vi "MainApp.vi"() -> ()   [LabVIEW 2018]
panel:
  out "Error Out":errorcluster
  in  "Plots":T1(tab)
  out "EEG":cluster{dbl[], dbl[]}(graph)
  out "PS":cluster{dbl[], dbl[]}(graph)
  out "Filtered":cluster{dbl[], dbl[]}(graph)
  in  "Save":bool
  in  "Filename":string
  out "Value":dbl
  out "State":T2(ring)
  in  "Stop":bool
  in  "Start":bool
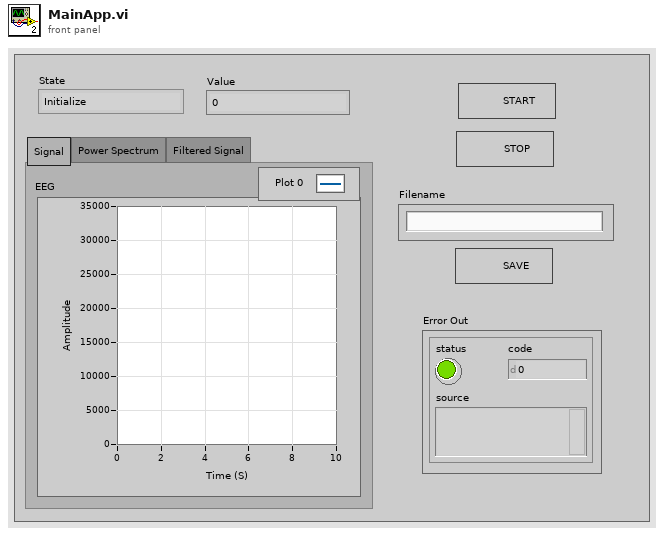
[diagram p1: front panel]
types:
  T1 = enum32{"Signal", "Power Spectrum", "Filtered Signal"}
  T2 = enum16{"Initialize", "Standby", "Record Data", "Filter Signal", "Save to File", "Stop"}
  T3 = enum16{"Standard", "Buffered", "CRLF", "Immediate"}
  T4 = enum16{"open", "replace", "create", "open or create", "replace or create", "replace or create with confirmation"}
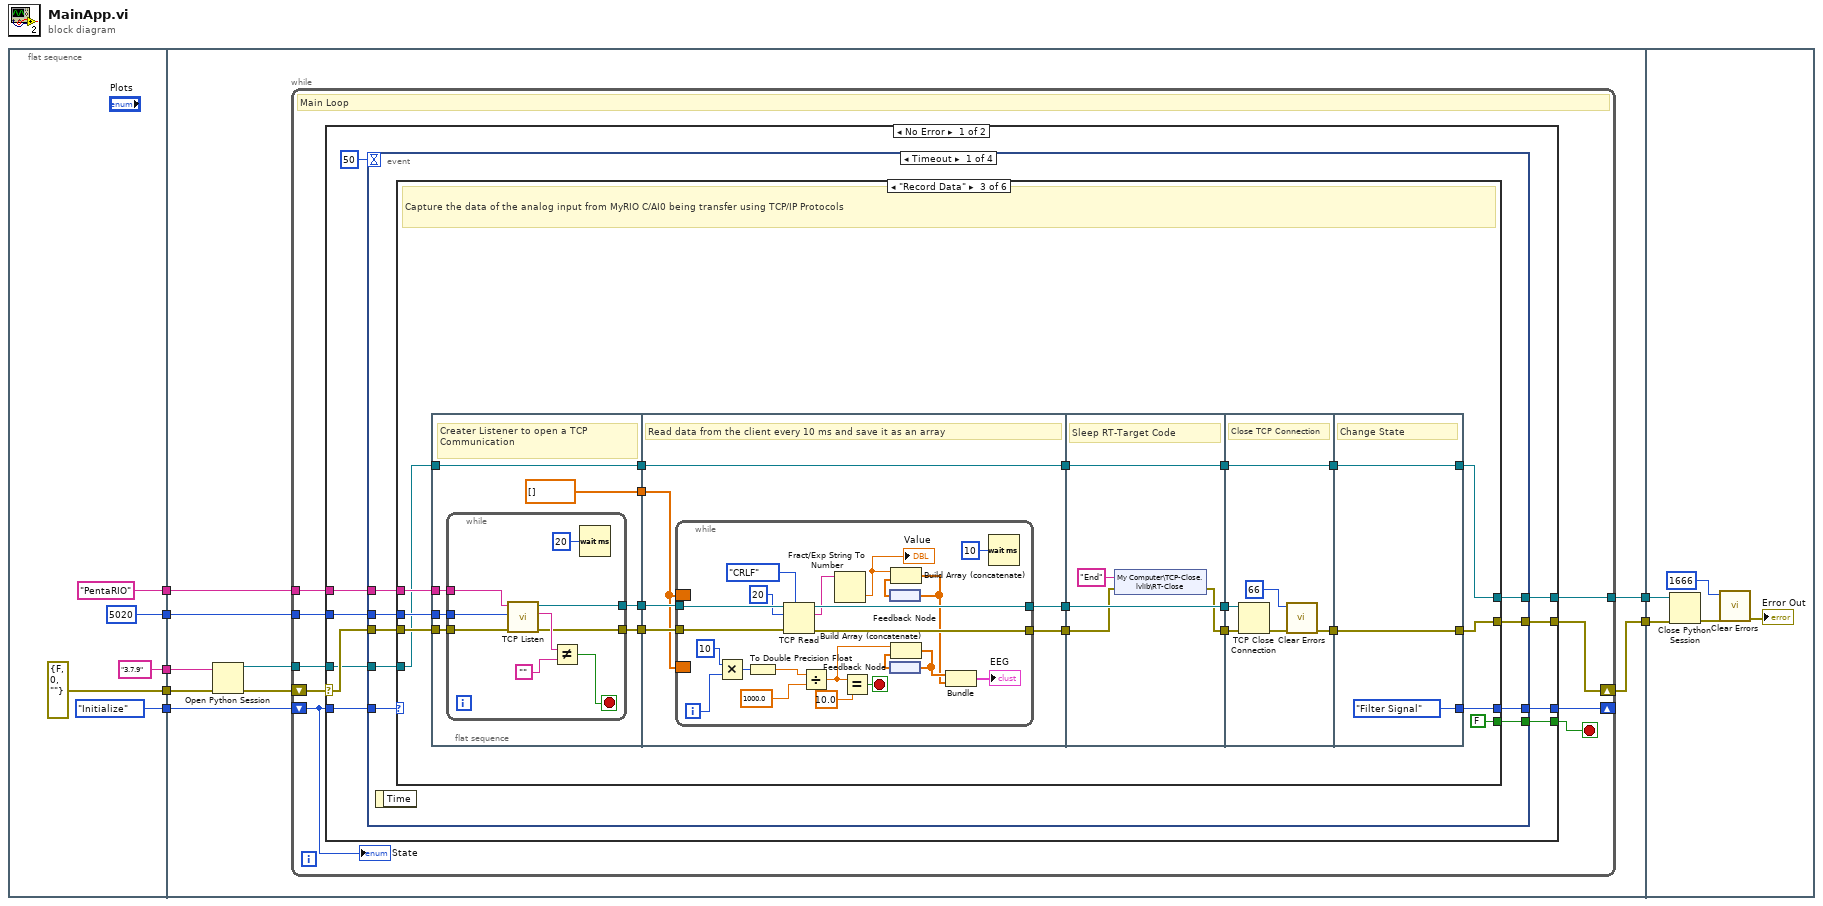
[diagram p0: block diagram]
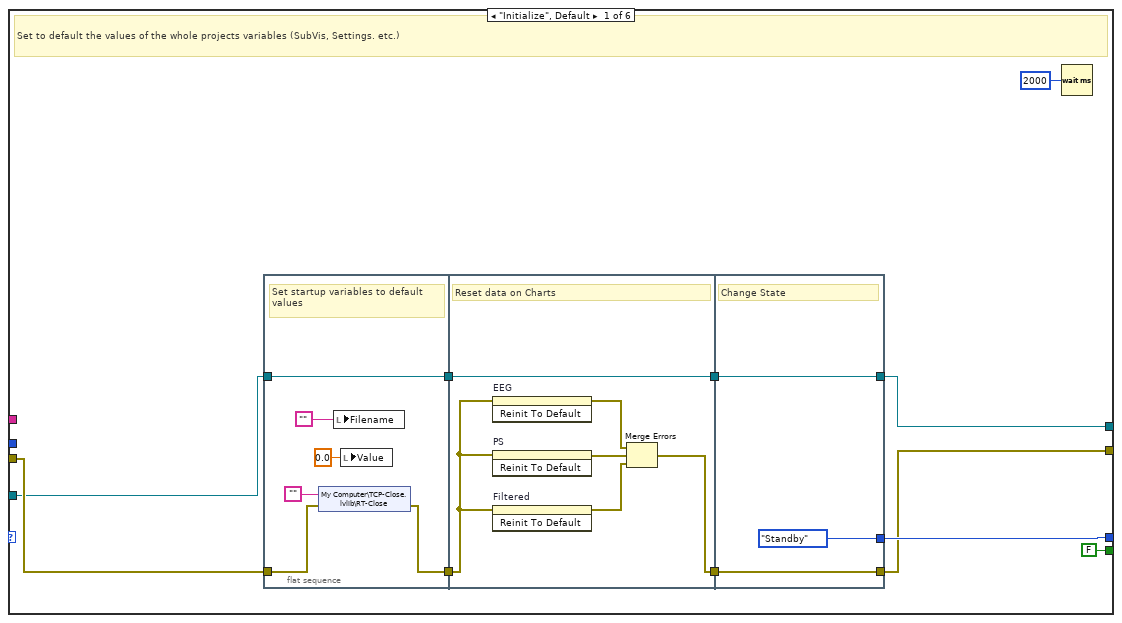
[diagram p2: hidden frame]
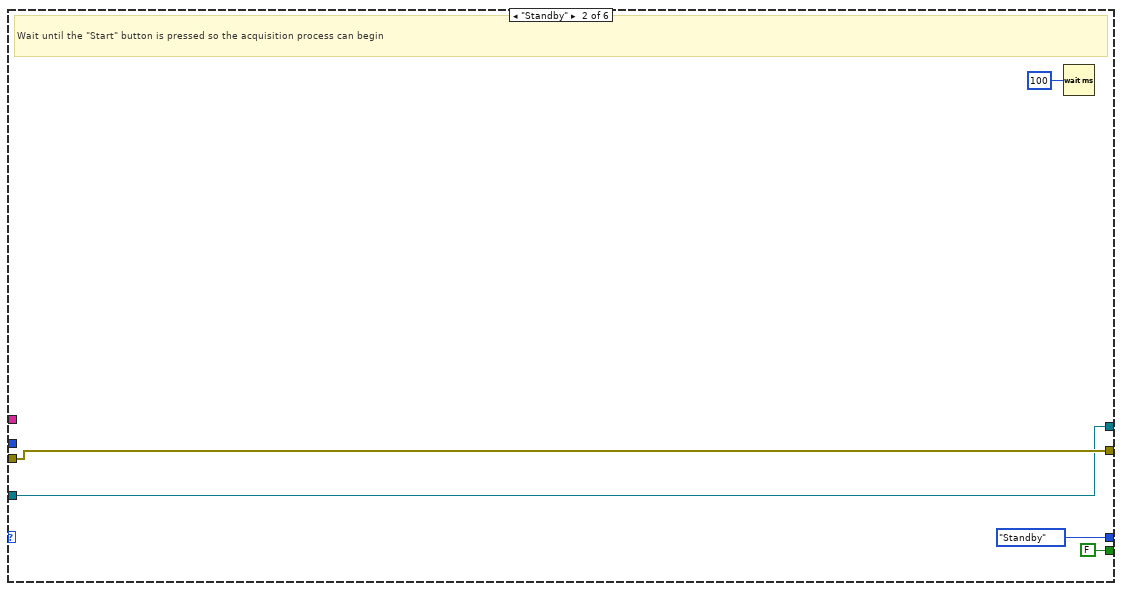
[diagram p3: hidden frame]
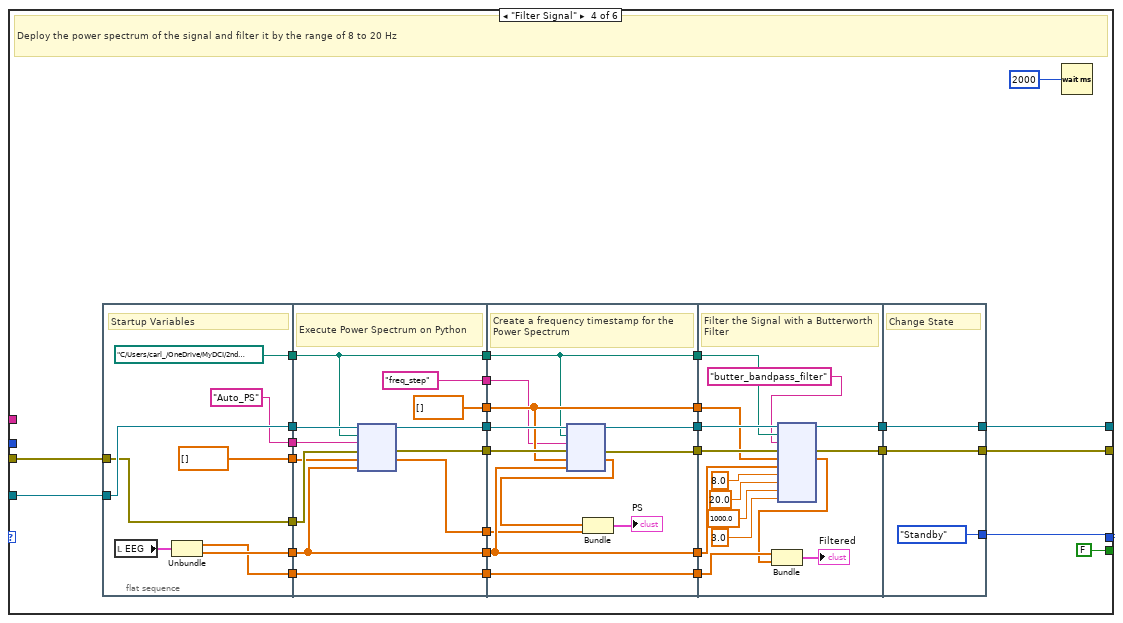
[diagram p4: hidden frame]
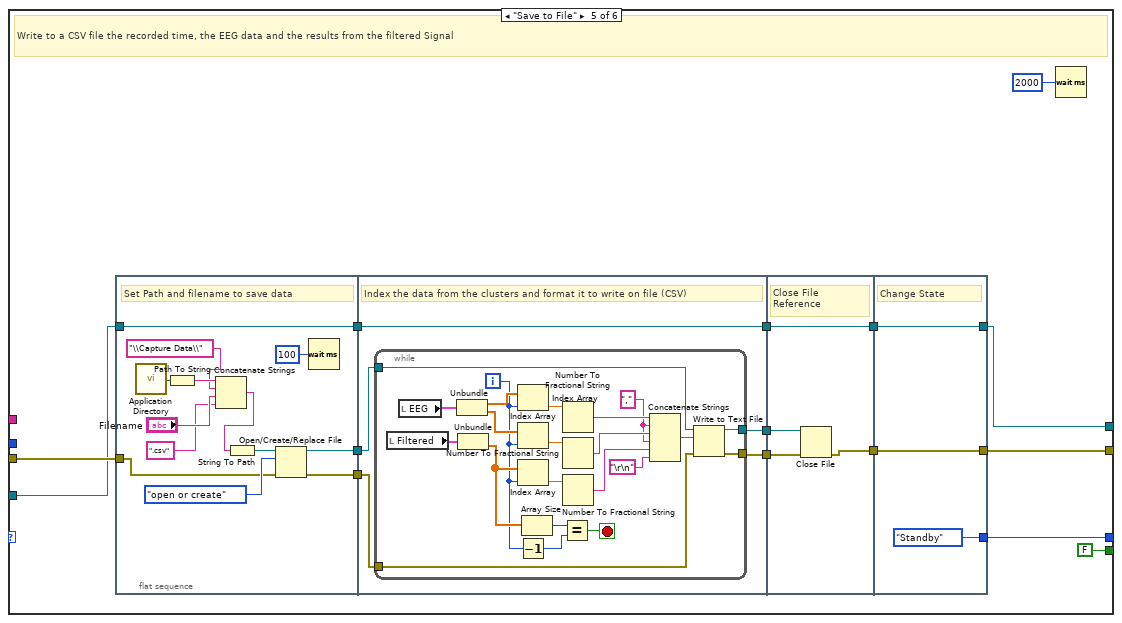
[diagram p5: hidden frame]
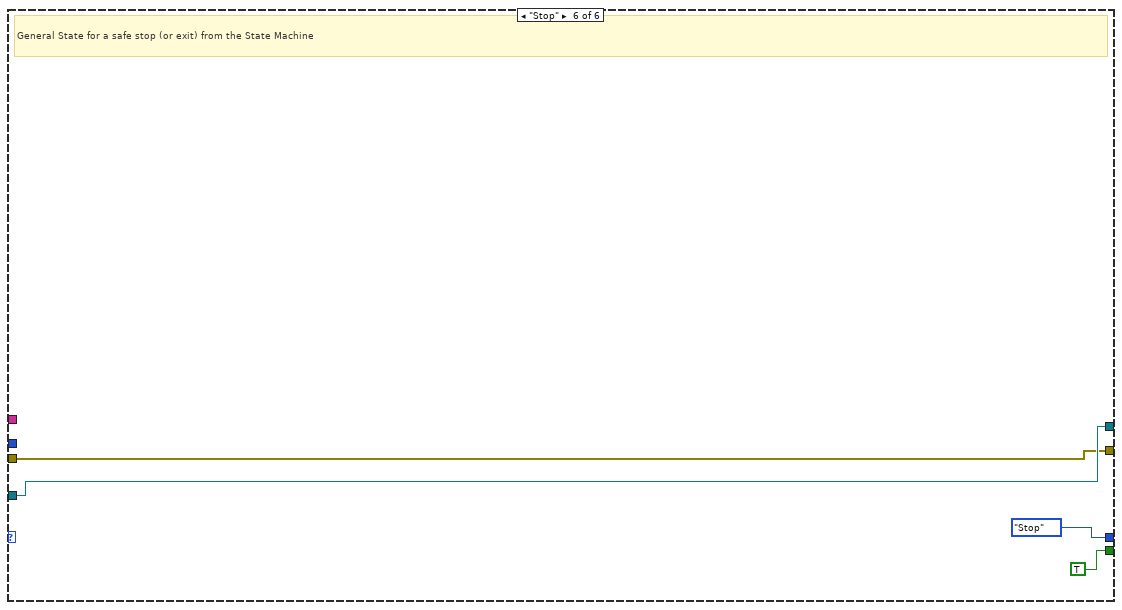
[diagram p6: hidden frame]
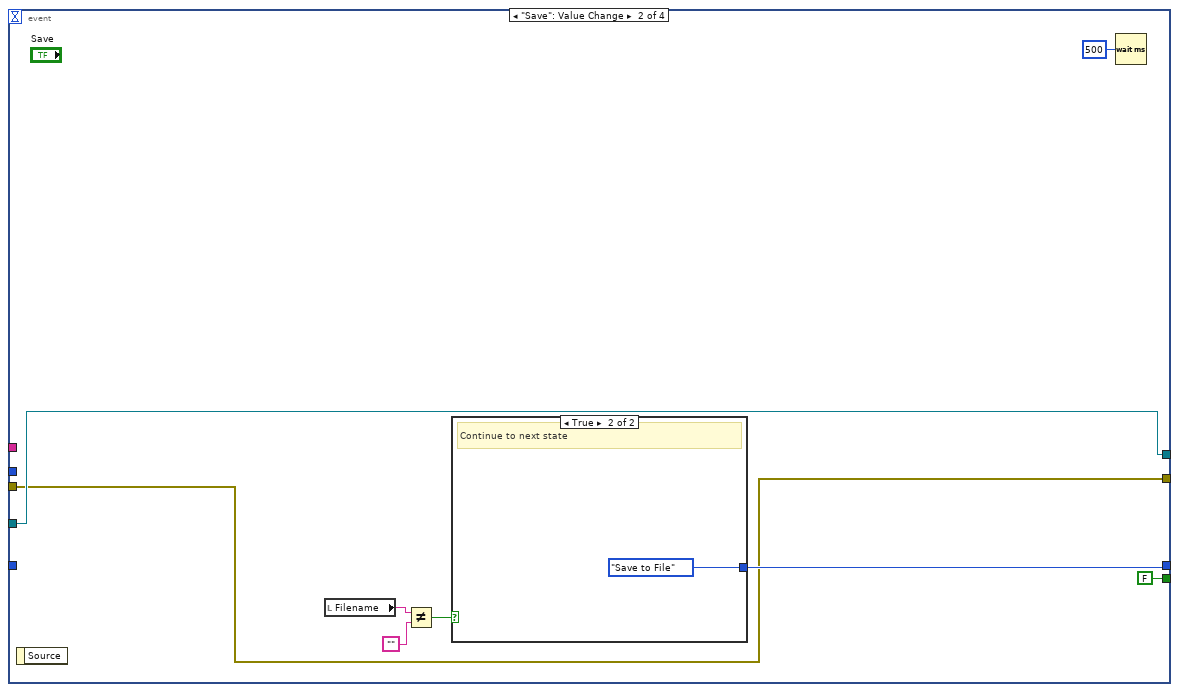
[diagram p7: hidden frame]
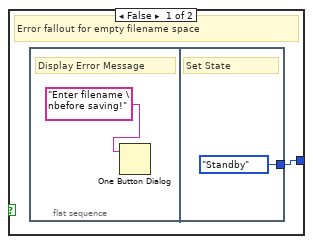
[diagram p8: hidden frame]
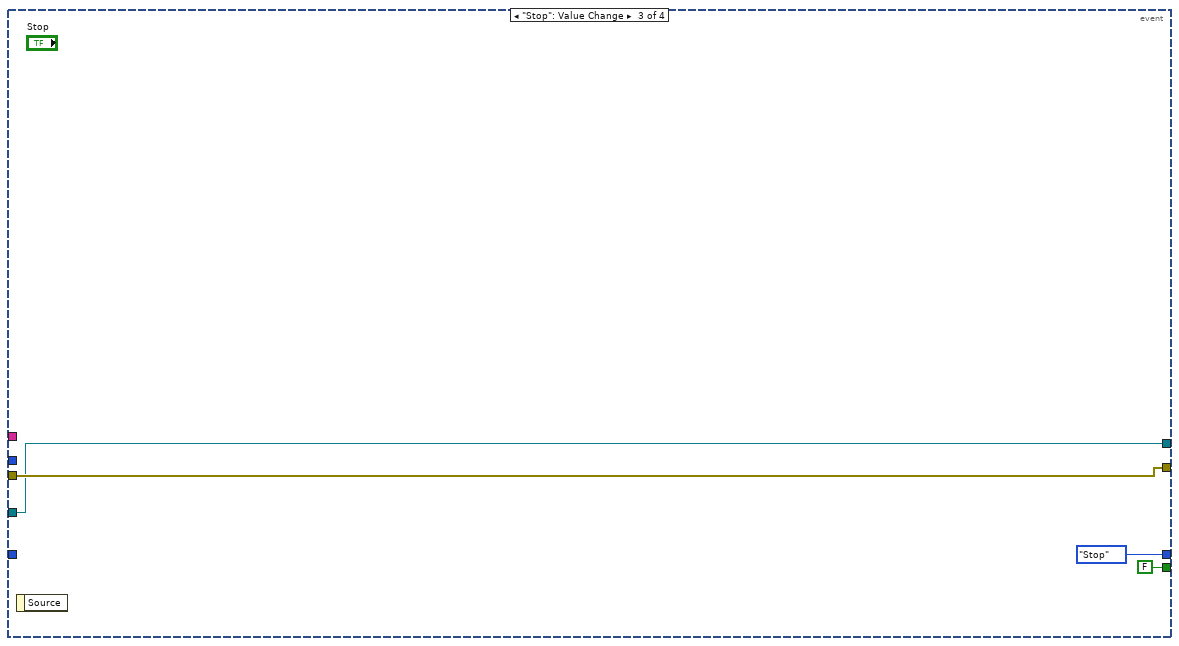
[diagram p9: hidden frame]
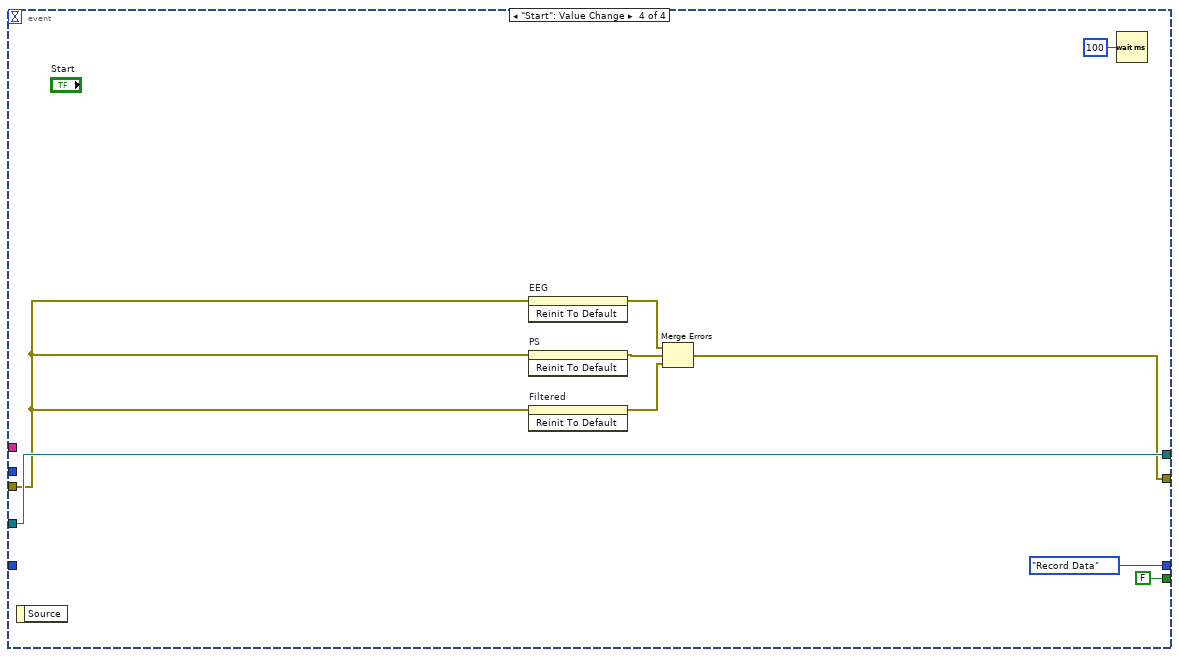
[diagram p10: hidden frame]
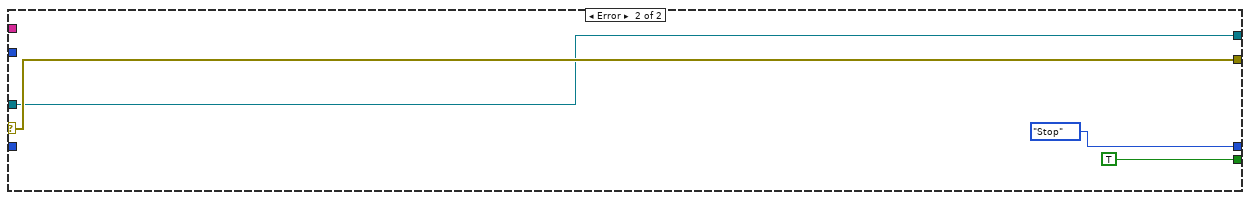
[diagram p11: hidden frame]
diagram:
  n1 = flat-sequence {
    tunnel: [T2."Initialize"] -> w7
    tunnel: [u16 5020 ("port")] -> w6
    tunnel: ["PentaRIO" ("service name")] -> w5
    tunnel: [errorcluster {"status"=FALSE, "code"=0, "source"=""} ("error constant")] -> w4
    tunnel: ["3.7.9" ("Python version")] -> w3
    tunnel: w7 -> [w21]
    tunnel: w6 -> [w20]
    tunnel: w5 -> [w19]
    tunnel: w4 -> [w18]
    tunnel: w3 -> [w16]
    tunnel: [w14] -> w2
    tunnel: [w13] -> w1
    tunnel: w2 -> [w338]
    tunnel: w1 -> [w337]
    frame #0 {
    }
    frame #1 {
      n2 = Open Python Session(python version=w16, 3:w18) -> (session out=w15:refnum<k35>, error out=w17:errorcluster)  [unwired: 1 in]
      n3 = while {
        shift-right: [w30] -> _
        shift-left: w21 -> [w29]
        tunnel: w20 -> [w28]
        tunnel: w19 -> [w27]
        tunnel: w15 -> [w25]
        tunnel: [w24] -> w14
        shift-right: [w23] -> w13
        shift-left: w17 -> [w26]
        stop <- w22 stop-if-true
        # "Main Loop"
        n4 = case shown="No Error" w26 {
          selector: w26 -> [w34 w332]
          tunnel: w29 -> [w39 _]
          tunnel: [w38 T2."Stop"] -> w30
          tunnel: [w37 TRUE] -> w22
          tunnel: w28 -> [w36 _]
          tunnel: w27 -> [w35 _]
          tunnel: w25 -> [w33 w331]
          tunnel: [w32 w331] -> w24
          tunnel: [w31 w332] -> w23
          frame No Error {
            n5 = event shown="[0] Timeout" {
              selector: _ -> [_ _ _ _]
              dyn-events: _ -> [_ _ _ _]
              timeout: 50 -> [_ _ _ _]
              tunnel: w39 -> [w49 _ _ _]
              tunnel: [w48 w308 T2."Stop" T2."Record Data"] -> w38
              tunnel: [w47 FALSE FALSE FALSE] -> w37
              tunnel: w34 -> [w46 w305 w318 w322]
              tunnel: w36 -> [w45 _ _ _]
              tunnel: w35 -> [w44 _ _ _]
              tunnel: w33 -> [w43 w306 w317 w327]
              tunnel: [w42 w306 w317 w327] -> w32
              tunnel: [w41 w305 w318 w325] -> w31
              event Timeout {
                n6 = event-data() -> ()  [unwired: 1 in, 1 out]
                n7 = case shown="\"Record Data\"" w49 {
                  tunnel: [w59 T2."Standby" w94 w161 w245 T2."Stop"] -> w48
                  tunnel: [FALSE FALSE FALSE FALSE FALSE TRUE] -> w47
                  tunnel: w46 -> [w57 w77 w100 w160 w252 w301]
                  tunnel: w45 -> [_ _ w99 _ _ _]
                  tunnel: w44 -> [_ _ w98 _ _ _]
                  tunnel: w43 -> [w54 w76 w90 w187 w243 w302]
                  tunnel: [w51 w76 w87 w179 w239 w302] -> w42
                  tunnel: [w55 w77 w91 w178 w247 w301] -> w41
                  frame "Initialize", Default {
                    # "Set to default the values of the whole projects variables (SubVis, Settings. etc.)"
                    n8 = flat-sequence {
                      tunnel: w57 -> [w62]
                      tunnel: w54 -> [w64]
                      tunnel: [w64] -> w52
                      tunnel: [w61] -> w50
                      tunnel: [w67] -> w56
                      tunnel: [w72] -> w53
                      tunnel: w52 -> [w72]
                      tunnel: w50 -> [w71]
                      tunnel: [T2."Standby"] -> w59
                      tunnel: [w74] -> w55
                      tunnel: w56 -> [w74]
                      tunnel: [w73] -> w51
                      tunnel: w53 -> [w73]
                      frame #0 {
                        # "Set startup variables to default values"
                        n9 = shared-variable "My Computer\\TCP-Close.lvlib\\RT-Close"("", error in=w62) -> (error out=w61:errorcluster)
                        n10 = local write "Filename"("") -> ()
                        n11 = local write "Value"(0.0 ("Value")) -> ()
                      }
                      frame #1 {
                        # "Reset data on Charts"
                        n12 = invoke on="EEG" class="XYGraph (strict)" method="Reinit To Default"(error in=w71) -> (error out=w70:errorcluster)  [unwired: 2 in, 2 out]
                        n13 = invoke on="PS" class="XYGraph (strict)" method="Reinit To Default"(error in=w71) -> (error out=w69:errorcluster)  [unwired: 2 in, 2 out]
                        n14 = invoke on="Filtered" class="XYGraph (strict)" method="Reinit To Default"(error in=w71) -> (error out=w68:errorcluster)  [unwired: 2 in, 2 out]
                        n15 = Merge Errors(w70, w69, w68) -> (w67:errorcluster)
                      }
                      frame #2 {
                        # "Change State"
                      }
                    }
                    n16 = Wait (ms)(milliseconds to wait=u32 2000) -> ()  [unwired: 1 out]
                  }
                  frame "Standby" {
                    # "Wait until the \"Start\" button is pressed so the acquisition process can begin"
                    n17 = Wait (ms)(milliseconds to wait=u32 100) -> ()  [unwired: 1 out]
                  }
                  frame "Record Data" {
                    # "Capture the data of the analog input from MyRIO C/AI0 being transfer using TCP/IP Protocols"
                    n18 = flat-sequence {
                      tunnel: w100 -> [w104]
                      tunnel: w99 -> [w103]
                      tunnel: w98 -> [w102]
                      tunnel: [w107] -> w97
                      tunnel: [w106] -> w96
                      tunnel: [dbl[] []] -> w95
                      tunnel: w90 -> [w101]
                      tunnel: [w101] -> w88
                      tunnel: w97 -> [w122]
                      tunnel: w96 -> [w121]
                      tunnel: w95 -> [w118]
                      tunnel: [w120] -> w86
                      tunnel: [w119] -> w84
                      tunnel: [w117] -> w82
                      tunnel: w88 -> [w117]
                      tunnel: w86 -> [w148]
                      tunnel: [w148] -> w85
                      tunnel: w84 -> [w146]
                      tunnel: [w145] -> w83
                      tunnel: w82 -> [w149]
                      tunnel: [w149] -> w81
                      tunnel: w85 -> [w154]
                      tunnel: w83 -> [w155]
                      tunnel: [w151] -> w93
                      tunnel: [w150] -> w89
                      tunnel: w81 -> [w150]
                      tunnel: [w158] -> w91
                      tunnel: w93 -> [w158]
                      tunnel: [T2."Filter Signal"] -> w94
                      tunnel: [w156] -> w87
                      tunnel: w89 -> [w156]
                      frame #0 {
                        # "Creater Listener to open a TCP Communication"
                        n19 = while {
                          tunnel: [w114] -> w107
                          tunnel: [w113] -> w106
                          tunnel: w104 -> [w110]
                          tunnel: w103 -> [w109]
                          tunnel: w102 -> [w108]
                          stop <- w115 stop-if-true
                          n20 = call <vilib>:"TCP Listen.vi"("error in (no error)"=w110, "port"=w109, "service name"=w108) -> ("error out"=w113:errorcluster, "remote address"=w116:string, "connection ID"=w114:refnum<k5>)  [unwired: 4 in, 2 out]
                          n21 = Not Equal?(x=w116, y="") -> (x != y?=w115:bool)
                          n22 = Wait (ms)(milliseconds to wait=u32 20) -> ()  [unwired: 1 out]
                        }
                      }
                      frame #1 {
                        # "Read data from the client every 10 ms and save it as an array"
                        n23 = while {
                          tunnel: w122 -> [w144]
                          tunnel: w121 -> [w143]
                          tunnel: [w140] -> w120
                          tunnel: [w139] -> w119
                          border: w118 -> [_]
                          border: w118 -> [_]
                          i -> [w137]
                          stop <- w134 stop-if-true
                          n24 = Multiply(x=10, y=w137) -> (x*y=w130:i32)
                          n25 = To Double Precision Float(number=w130) -> (double precision float=w129:dbl)
                          n26 = TCP Read(connection ID=w144, bytes to read=20, error in (no error)=w143, 7:T3."CRLF" ("mode (standard)")) -> (connection ID out=w140:refnum<k5>, data out=w133:string, error out=w139:errorcluster)  [unwired: 1 in]
                          n27 = Divide(x=w129, y=1000.0) -> (x/y=w127:dbl)
                          n28 = Fract/Exp String To Number(string=w133) -> (number=w131:dbl)  [unwired: 3 in, 1 out]
                          "Value" <- w131
                          n29 = Equal?(x=w127, y=10.0) -> (x = y?=w134:bool)
                          n30 = feedback #1() -> (w132:dbl[])
                          n31 = feedback #2() -> (w126:dbl[])
                          n32 = Build Array (concatenate)(w131, w132) -> (w124:dbl[])
                          n33 = feedback-in #1(w124) -> ()
                          n34 = Build Array (concatenate)(w127, w126) -> (w125:dbl[])
                          n35 = feedback-in #2(w125) -> ()
                          n36 = Bundle(w125, w124) -> (→"EEG":cluster{dbl[], dbl[]})  [unwired: 1 in]
                          n37 = Wait (ms)(milliseconds to wait=u32 10) -> ()  [unwired: 1 out]
                        }
                      }
                      frame #2 {
                        # "Sleep RT-Target Code"
                        n38 = shared-variable "My Computer\\TCP-Close.lvlib\\RT-Close"("End" ("RT-Close"), error in=w146) -> (error out=w145:errorcluster)
                      }
                      frame #3 {
                        # "Close TCP Connection"
                        n39 = TCP Close Connection(connection ID=w154, error in (no error)=w155) -> (error out=w153:errorcluster)  [unwired: 1 in, 1 out]
                        n40 = call <vilib>:"Clear Errors.vi"("error in (no error)"=w153, "specific error code to clear (0: all)"=66) -> ("error out"=w151:errorcluster)  [unwired: 4 in, 1 out]
                      }
                      frame #4 {
                        # "Change State"
                      }
                    }
                  }
                  frame "Filter Signal" {
                    # "Deploy the power spectrum of the signal and filter it by the range of 8 to 20 Hz"
                    n41 = flat-sequence {
                      tunnel: w187 -> [w195]
                      tunnel: [w189] -> w186
                      tunnel: [w195] -> w185
                      tunnel: [path "C:/Users/carl_/OneDrive/MyDCI/2nd Semester/Procesamiento Digital de Senales con Instrumentacion Virtual/EEG/EEG Integration/Filtering-Python37.py" ("module path")] -> w184
                      tunnel: [dbl[] []] -> w183
                      tunnel: [w192] -> w182
                      tunnel: [w191] -> w181
                      tunnel: ["Auto_PS" ("function name")] -> w180
                      tunnel: w160 -> [w189]
                      tunnel: w186 -> [w203]
                      tunnel: w185 -> [w206]
                      tunnel: w184 -> [w201]
                      tunnel: w183 -> [w202]
                      tunnel: w182 -> [w200]
                      tunnel: [w205] -> w177
                      tunnel: [w201] -> w175
                      tunnel: [dbl[] []] -> w173
                      tunnel: [w200] -> w171
                      tunnel: [w207] -> w169
                      tunnel: w181 -> [w207]
                      tunnel: w180 -> [w199]
                      tunnel: [w204] -> w167
                      tunnel: [w198] -> w165
                      tunnel: ["freq_step" ("function name")] -> w164
                      tunnel: w177 -> [w219]
                      tunnel: [w217] -> w176
                      tunnel: w175 -> [w214]
                      tunnel: [w214] -> w174
                      tunnel: w173 -> [w215]
                      tunnel: [w215] -> w172
                      tunnel: w171 -> [w213]
                      tunnel: [w213] -> w170
                      tunnel: w169 -> [w220]
                      tunnel: [w220] -> w168
                      tunnel: w167 -> [w218]
                      tunnel: [w216] -> w166
                      tunnel: w165 -> [w210]
                      tunnel: w164 -> [w211]
                      tunnel: w176 -> [w235]
                      tunnel: w174 -> [w231]
                      tunnel: w172 -> [w230]
                      tunnel: w170 -> [w228]
                      tunnel: w168 -> [w223]
                      tunnel: w166 -> [w234]
                      tunnel: [w233] -> w163
                      tunnel: [w232] -> w162
                      tunnel: [w237] -> w178
                      tunnel: [w238] -> w179
                      tunnel: w163 -> [w238]
                      tunnel: w162 -> [w237]
                      tunnel: [T2."Standby"] -> w161
                      frame #0 {
                        # "Startup Variables"
                        n42 = local read "EEG"() -> (w196:cluster{dbl[], dbl[]})
                        n43 = Unbundle(w196) -> (w191:dbl[], w192:dbl[])
                      }
                      frame #1 {
                        # "Execute Power Spectrum on Python"
                        n44 = node(w206, w201, w199, w203, w202, w200) -> (w205:refnum<k35>, w204:errorcluster, w198:dbl[])  [unwired: 1 in, 2 out]
                      }
                      frame #2 {
                        # "Create a frequency timestamp for the Power Spectrum"
                        n45 = node(w219, w214, w211, w218, w215, w213) -> (w217:refnum<k35>, w216:errorcluster, w209:dbl[])  [unwired: 1 in, 2 out]
                        n46 = Bundle(w209, w210) -> (→"PS":cluster{dbl[], dbl[]})  [unwired: 1 in]
                      }
                      frame #3 {
                        # "Filter the Signal with a Butterworth Filter"
                        n47 = node(w235, w231, "butter_bandpass_filter" ("function name"), w234, w230, w228, 8.0, 20.0, 1000.0, 3.0) -> (w233:refnum<k35>, w232:errorcluster, w222:dbl[])  [unwired: 5 in, 2 out]
                        n48 = Bundle(w223, w222) -> (→"Filtered":cluster{dbl[], dbl[]})  [unwired: 1 in]
                      }
                      frame #4 {
                        # "Change State"
                      }
                    }
                    n49 = Wait (ms)(milliseconds to wait=u32 2000) -> ()  [unwired: 1 out]
                  }
                  frame "Save to File" {
                    # "Write to a CSV file the recorded time, the EEG data and the results from the filtered Signal"
                    n50 = flat-sequence {
                      tunnel: w252 -> [w260]
                      tunnel: [w266] -> w251
                      tunnel: [w265] -> w250
                      tunnel: w243 -> [w254]
                      tunnel: [w254] -> w240
                      tunnel: w251 -> [w271]
                      tunnel: w250 -> [w270]
                      tunnel: [w269] -> w249
                      tunnel: [w268] -> w248
                      tunnel: [w267] -> w241
                      tunnel: w240 -> [w267]
                      tunnel: w249 -> [w297]
                      tunnel: w248 -> [w296]
                      tunnel: [w295] -> w246
                      tunnel: [w294] -> w242
                      tunnel: w241 -> [w294]
                      tunnel: [w300] -> w247
                      tunnel: w246 -> [w300]
                      tunnel: [T2."Standby"] -> w245
                      tunnel: [w298] -> w239
                      tunnel: w242 -> [w298]
                      frame #0 {
                        # "Set Path and filename to save data"
                        n51 = call <vilib>:"Application Directory.vi"() -> ("Application Directory"=w261:path)
                        n52 = Path To String(path=w261) -> (string=w256:string)
                        n53 = Concatenate Strings(w256, "\\Capture Data\\", "Filename", ".csv" ("string")) -> (w263:string)
                        n54 = String To Path(string=w263) -> (path=w264:path)
                        n55 = Open/Create/Replace File(file path (use dialog)=w264, error in=w260, operation (0:open)=T4."open or create") -> (refnum out=w266:refnum<file>, error out=w265:errorcluster)  [unwired: 3 in, 1 out]
                        n56 = Wait (ms)(milliseconds to wait=u32 100) -> ()  [unwired: 1 out]
                      }
                      frame #1 {
                        # "Index the data from the clusters and format it to write on file (CSV)"
                        n57 = while {
                          tunnel: w271 -> [w275]
                          tunnel: w270 -> [w274]
                          tunnel: [w273] -> w269
                          tunnel: [w272] -> w268
                          i -> [w277]
                          stop <- w279 stop-if-true
                          w284 = "," ("string")
                          n58 = local read "Filtered"() -> (w292:cluster{dbl[], dbl[]})
                          n59 = local read "EEG"() -> (w293:cluster{dbl[], dbl[]})
                          n60 = Unbundle(w293) -> (w291:dbl[], w290:dbl[])
                          n61 = Unbundle(w292) -> (w281:dbl[])  [unwired: 1 out]
                          n62 = Index Array(array=w291, index=w277) -> (element=w289:dbl)
                          n63 = Index Array(array=w290, index=w277) -> (element=w287:dbl)
                          n64 = Index Array(array=w281, index=w277) -> (element=w288:dbl)
                          n65 = Decrement(x=w277) -> (x-1=w278:i32)
                          n66 = Array Size(array=w281) -> (size(s)=w280:i32)
                          n67 = Equal?(x=w280, y=w278) -> (x = y?=w279:bool)
                          n68 = Number To Fractional String(number=w289) -> (F-format string=w286:string)  [unwired: 3 in]
                          n69 = Number To Fractional String(number=w287) -> (F-format string=w285:string)  [unwired: 3 in]
                          n70 = Number To Fractional String(number=w288) -> (F-format string=w283:string)  [unwired: 3 in]
                          n71 = Concatenate Strings(w286, w284, w285, w284, w283, "\r\n") -> (w276:string)
                          n72 = Write to Text File(file (use dialog)=w275, text=w276, error in=w274) -> (refnum out=w273:refnum<file>, error out=w272:errorcluster)  [unwired: 1 in, 1 out]
                        }
                      }
                      frame #2 {
                        # "Close File Reference"
                        n73 = Close File(refnum=w297, error in=w296) -> (error out=w295:errorcluster)  [unwired: 1 out]
                      }
                      frame #3 {
                        # "Change State"
                      }
                    }
                    n74 = Wait (ms)(milliseconds to wait=u32 2000) -> ()  [unwired: 1 out]
                  }
                  frame "Stop" {
                    # "General State for a safe stop (or exit) from the State Machine"
                  }
                }
              }
              event "Save": Value Change {
                n75 = event-data() -> ()  [unwired: 1 in, 1 out]
                n76 = local read "Filename"() -> (w311:string)
                n77 = Not Equal?(x=w311, y="") -> (x != y?=w309:bool)
                n78 = case shown="True" w309 {
                  tunnel: [w313 T2."Save to File"] -> w308
                  frame False {
                    # "Error fallout for empty filename space"
                    n79 = flat-sequence {
                      tunnel: [T2."Standby"] -> w313
                      frame #0 {
                        # "Display Error Message"
                        n80 = One Button Dialog(message="Enter filename \nbefore saving!") -> ()  [unwired: 1 in, 1 out]
                      }
                      frame #1 {
                        # "Set State"
                      }
                    }
                  }
                  frame True {
                    # "Continue to next state"
                  }
                }
                n81 = Wait (ms)(milliseconds to wait=u32 500) -> ()  [unwired: 1 out]
              }
              event "Stop": Value Change {
                n82 = event-data() -> ()  [unwired: 1 in, 1 out]
              }
              event "Start": Value Change {
                n83 = event-data() -> ()  [unwired: 1 in, 1 out]
                n84 = invoke on="EEG" class="XYGraph (strict)" method="Reinit To Default"(error in=w322) -> (error out=w324:errorcluster)  [unwired: 2 in, 2 out]
                n85 = invoke on="PS" class="XYGraph (strict)" method="Reinit To Default"(error in=w322) -> (error out=w323:errorcluster)  [unwired: 2 in, 2 out]
                n86 = invoke on="Filtered" class="XYGraph (strict)" method="Reinit To Default"(error in=w322) -> (error out=w321:errorcluster)  [unwired: 2 in, 2 out]
                n87 = Merge Errors(w324, w323, w321) -> (w325:errorcluster)
                n88 = Wait (ms)(milliseconds to wait=u32 100) -> ()  [unwired: 1 out]
              }
            }
          }
          frame Error {
          }
        }
        "State" <- w29
      }
    }
    frame #2 {
      n89 = Close Python Session(session in=w338, error in=w337) -> (11:w336:errorcluster)
      n90 = call <vilib>:"Clear Errors.vi"("error in (no error)"=w336, "specific error code to clear (0: all)"=1666) -> ("error out"=→"Error Out":errorcluster)  [unwired: 4 in, 1 out]
    }
  }
